vi "Change Control Reference.vi"(8 "error in":errorcluster, 10 "Reference In":variant, 11 "BigMAQ in":refnum<class "BigMAQ.lvclass">) -> (0 "error out":errorcluster, 1 "Image Control":T1, 3 "BigMAQ out":refnum<class "BigMAQ.lvclass">)   [LabVIEW 2019, in "BigMAQ.lvclass"]
uses:
  BigMAQ.lvclass
  <vilib>/vision/Image Controls.llb/IMAQ Image.ctl
  BigMAQ.lvclass/BigMAQ.ctl
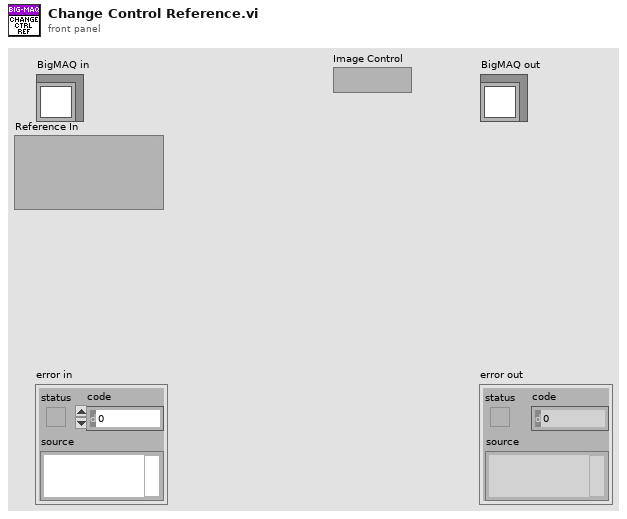
[diagram p1: front panel]
types:
  T1 = typedef "IMAQ Image.ctl" = refnum<image>
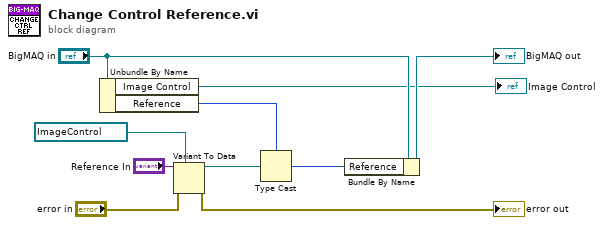
[diagram p0: block diagram]
diagram:
  n1 = Unbundle By Name("BigMAQ in") -> ("Image Control"=→"Image Control":T1, "Reference"=w8:i32)
  n2 = Variant To Data(error in="error in", type=refnum<vi> refnum ("reference"), Variant="Reference In") -> (data=w7:refnum<vi>, error out=→"error out":errorcluster)
  n3 = Type Cast(type=w8, x=w7) -> (*(type *) &x=w6:i32)
  n4 = Bundle By Name(cluster="BigMAQ in", "Reference"=w6) -> (→"BigMAQ out":refnum<class "BigMAQ.lvclass">)
